vi "Main.vi"(11 "Module Admin":refnum<class "Delacor_lib_QMH_Module Admin.lvclass">) -> ()   [LabVIEW 2020, in "My Singleton Module.lvlib"]
doc: "This template is based off of the Queued Message Handler design pattern and the Queued Message Handler project template that ships with LabVIEW.\n\nThe main difference is that the queue is private to this module and communication between modules is performed via Broadcast and Request events.\n\nRequest events are wrapped in public API methods and are handled in the Event Handling Loop (EHL) of this VI. Any module can register for Broadcast events sent by this module. The EHL generates messages based on user interface actions.\n\nThe Message Handling Loop (MHL) processes messages generated by the EHL, or by other messages. The messages are string values, so new messages can be added easily to the Message Cases case structure in the MHL. Each message cluster can also provide an optional value for Message Data, which is a variant that can be converted to whatever message-specific data is required.\n_____\nBased on Delacor QMH Project Template 5.0.0.82."
uses:
  My Singleton Module.lvlib
  <vilib>/Delacor/Delacor QMH/Libraries/Module Admin_class/Delacor_lib_QMH_Module Admin.lvclass
  Module Data--cluster.ctl
  Do Something Argument--cluster.ctl
  <vilib>/Delacor/Delacor QMH/Libraries/Message Queue_class/Delacor_lib_QMH_Message Queue.lvclass/Delacor_lib_QMH_Message Queue.ctl
  Do Something Else Argument--cluster.ctl
  Do Something Else and Wait for Reply Argument--cluster.ctl
  Do Something Else and Wait (Reply Payload)--cluster.ctl
  Stop Argument--cluster.ctl
  <vilib>/Delacor/Delacor QMH/Libraries/Module Admin_class/Delacor_lib_QMH_Module Admin.lvclass/Delacor_lib_QMH_Module Admin.ctl
  <vilib>/Utility/miscctls.llb/LVPointTypeDef.ctl
  <vilib>/Delacor/Delacor QMH/Libraries/Message Queue_class/Delacor_lib_QMH_Enqueue Message (Single).vi
  <vilib>/Delacor/Delacor QMH/Libraries/Module Admin_class/Delacor_lib_QMH_Get External Launch.vi
  <vilib>/Utility/error.llb/Error Cluster From Error Code.vi
  <vilib>/ErrorRing/Error Ring.xnode
  <vilib>/Delacor/Delacor QMH/Libraries/Message Queue_class/Delacor_lib_QMH_Message Queue.lvclass
panel:
  in  "Simulate MHL Error":bool
  in  "Simulate EHL Error":bool
  out "error out":errorcluster
  out "X":dbl
  out "Status":string
  in  "Do Something Else <Replace Me>":bool
  in  "Do Something <Replace Me>":bool
  # "These controls have associated \"Value Changed\" events configured in the Event Structure on the diagram.\n\nReplace them (and reconfigure the Event Structure) with the controls you need for your application. \n\nOther QMH Modules communicate with this Module via its Public API (wrappers for its Request Events).\n\nThis Module communicates with other Modules via its Broadcast Events.\nAny module that wants to get these messages, just registers for this module's Broadcast events."
  # "This template is for the Delacor Modified Queued Message Handler design pattern.\n\nSee the block diagram for more information on how to use this template."
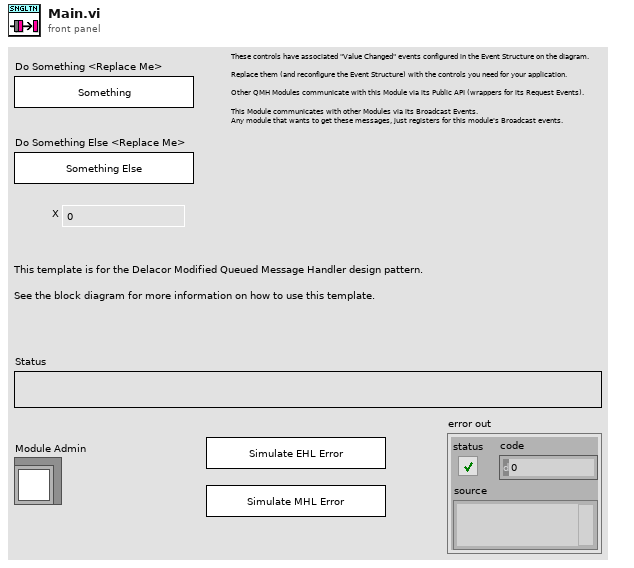
[diagram p1: front panel]
types:
  T1 = typedef "My Singleton Module.lvlib/Request Events--cluster.ctl" = cluster{"Stop Module":refnum<user-event>, "Do Something":refnum<user-event>, "Do Something Else":refnum<user-event>, "Do Something Else and Wait for Reply":refnum<user-event>, "Show Panel":refnum<user-event>, "Hide Panel":refnum<user-event>, "Get Module Execution Status":refnum<user-event>, "Show Diagram":refnum<user-event>}
  T2 = typedef "My Singleton Module.lvlib/Module Data--cluster.ctl" = cluster{"Status":string}
  T3 = typedef "My Singleton Module.lvlib/Do Something Argument--cluster.ctl" = cluster{"Do Something Msg":string}
  T4 = typedef "My Singleton Module.lvlib/Do Something Else Argument--cluster.ctl" = cluster{"Do Something Else Msg":string, "X":dbl}
  T5 = typedef "My Singleton Module.lvlib/Do Something Else and Wait for Reply Argument--cluster.ctl" = cluster{"Do Something Else Msg":string, "X":dbl, "Wait Notifier":refnum<notifier>, "wait for reply":bool}
  T6 = enum32{"invalid lock state", "Not Locked", "Locked (No Password)", "Password-protected"}
  T7 = typedef "My Singleton Module.lvlib/Stop Argument--cluster.ctl" = cluster{"Origin":string, "Exit via Stop Module Req?":bool, "Wait for Module to stop?":bool}
  T8 = typedef "LVPointTypeDef.ctl" = cluster{"Horizontal":i16, "Vertical":i16}
  T9 = enum32{"Invalid", "Standard", "Closed", "Hidden", "Minimized", "Maximized"}
  T10 = typedef "My Singleton Module.lvlib/Do Something Else and Wait (Reply Payload)--cluster.ctl" = cluster{"Value":dbl, "error":errorcluster}
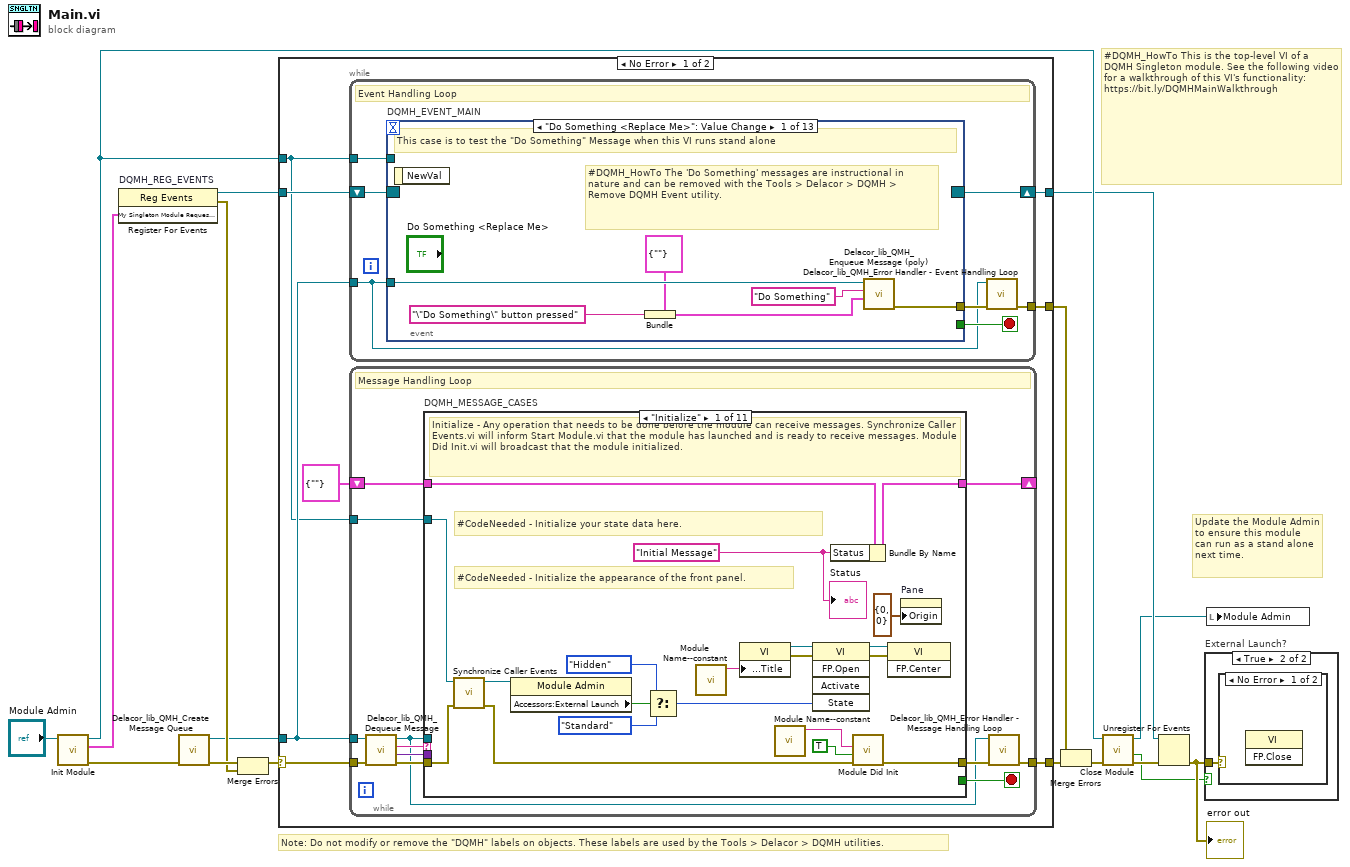
[diagram p0: block diagram]
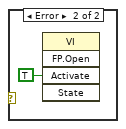
[diagram p3: hidden frame]
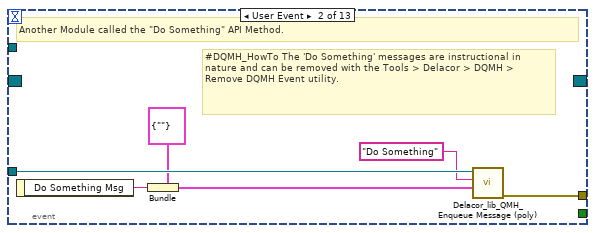
[diagram p4: hidden frame]
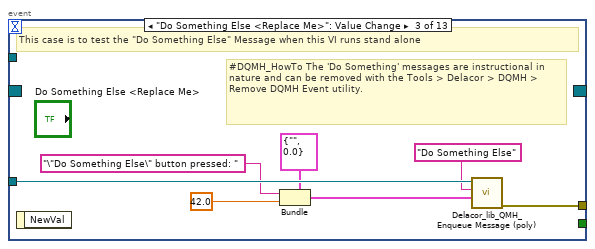
[diagram p5: hidden frame]
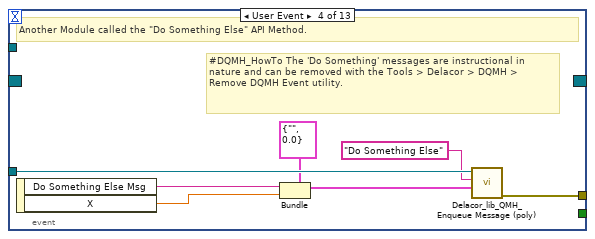
[diagram p6: hidden frame]
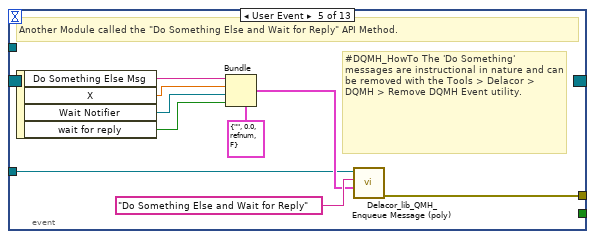
[diagram p7: hidden frame]
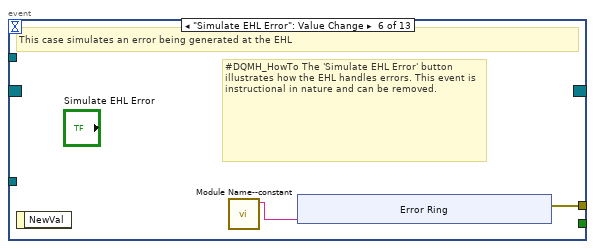
[diagram p8: hidden frame]
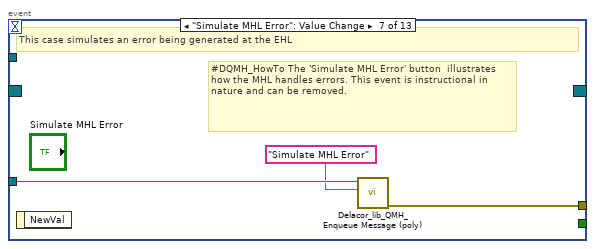
[diagram p9: hidden frame]
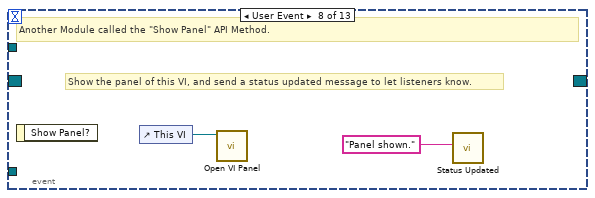
[diagram p10: hidden frame]
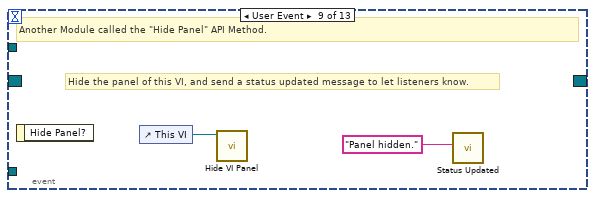
[diagram p11: hidden frame]
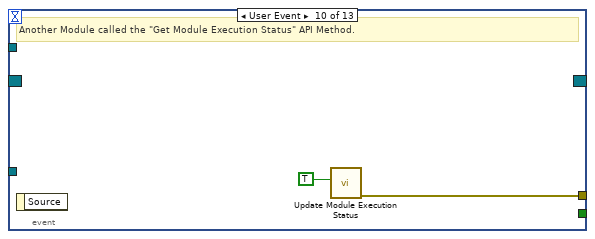
[diagram p12: hidden frame]
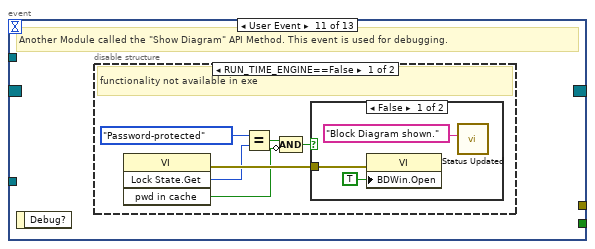
[diagram p13: hidden frame]
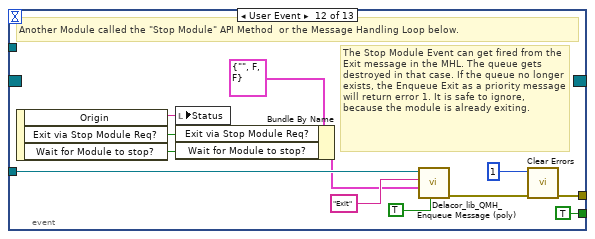
[diagram p16: hidden frame]
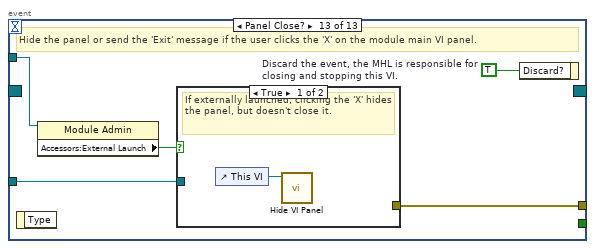
[diagram p17: hidden frame]
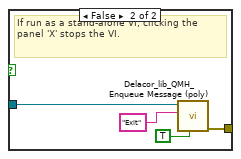
[diagram p18: hidden frame]
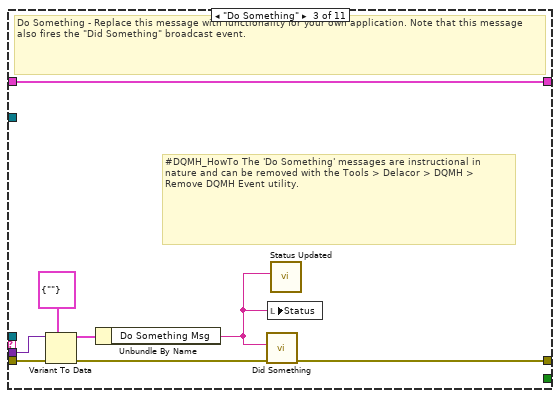
[diagram p20: hidden frame]
diagram:
  # "#DQMH_HowTo This is the top-level VI of a DQMH Singleton module. See the following video for a walkthrough of this VI's functionality: https://bit.ly/DQMHMainWalkthrough"
  # "Note: Do not modify or remove the \"DQMH\" labels on objects. These labels are used by the Tools > Delacor > DQMH utilities."
  # "Update the Module Admin to ensure this module can run as a stand alone next time."
  n1 = call "Init Module.vi"("Singleton Module Admin in"="Module Admin") -> ("error out"=w16:errorcluster, "My Singleton Module Request Events"=w5:T1, "Singleton Module Admin out"=w8:refnum<class "Delacor_lib_QMH_Module Admin.lvclass">)  [unwired: 8 in]
  n2 = register-events "DQMH_REG_EVENTS"(w5) -> (reference out=w6:refnum<event-registration>, error out=w9:errorcluster)  [unwired: 2 in]
  n3 = call <vilib>:"Delacor_lib_QMH_Create Message Queue.vi"("error in (no error)"=w16) -> ("error out"=w11:errorcluster, "Message Queue"=w4:refnum<class "Delacor_lib_QMH_Message Queue.lvclass">)  [unwired: 9 in]
  n4 = Merge Errors(w11, w9) -> (w10:errorcluster)
  n5 = case shown="No Error" w10 {
    selector: w10 -> [w23 w264]
    tunnel: [w25 w263] -> w17
    tunnel: [w22 w269] -> w7
    tunnel: w6 -> [w20 w269]
    tunnel: w4 -> [w19 w262]
    tunnel: [w24 _] -> w14
    tunnel: w8 -> [w18 w265]
    frame No Error {
      n6 = while {
        tunnel: w19 -> [w26]
        shift-right: [w29] -> w22
        shift-left: w20 -> [w30]
        tunnel: [w31] -> w24
        tunnel: w18 -> [w27]
        stop <- w28 stop-if-true
        # "Event Handling Loop"
        n7 = event "DQMH_EVENT_MAIN" shown="[0] \"Do Something <Replace Me>\": Value Change" {
          selector: w30 -> [_ _ _ _ _ _ _ _ _ _ _ _ _]
          dyn-events: [_ _ _ _ _ _ _ _ _ _ _ _ _] -> w29
          timeout: _ -> [_ _ _ _ _ _ _ _ _ _ _ _ _]
          tunnel: [_ _ _ _ _ _ _ _ _ _ _ TRUE ("Discard?") _] -> w28
          tunnel: w26 -> [w37 w43 w50 w57 w60 _ w78 _ _ _ _ w102 w109]
          tunnel: [w38 w44 w51 w58 w67 w69 w79 _ _ w85 _ w105 w111] -> w32
          tunnel: w27 -> [_ _ _ _ _ _ _ _ _ _ _ _ w108]
          event "Do Something <Replace Me>": Value Change {
            # "#DQMH_HowTo The 'Do Something' messages are instructional in nature and can be removed with the Tools > Delacor > DQMH > Remove DQMH Event utility."
            # "This case is to test the \"Do Something\" Message when this VI runs stand alone"
            n8 = event-data() -> ()  [unwired: 1 in, 1 out]
            n9 = Bundle(cluster=T3 {"Do Something Msg"=""} ("Do Something Argument"), "Do Something Msg"="\"Do Something\" button pressed" ("\"Do Something\" button pressed")) -> (w33:T3)
            n10 = call-poly <vilib>:"Delacor_lib_QMH_Enqueue Message (poly).vi"("Message Data"=w33, "Message"="Do Something", "Message Queue in"=w37) -> ("error out"=w38:errorcluster)  [unwired: 7 in, 1 out]
          }
          event User Event {
            # "#DQMH_HowTo The 'Do Something' messages are instructional in nature and can be removed with the Tools > Delacor > DQMH > Remove DQMH Event utility."
            # "Another Module called the \"Do Something\" API Method."
            n11 = event-data() -> ("Do Something Msg"=w40:string)  [unwired: 1 in]
            n12 = Bundle(cluster=T3 {"Do Something Msg"=""} ("Do Something Argument"), "Do Something Msg"=w40) -> (w39:T3)
            n13 = call-poly <vilib>:"Delacor_lib_QMH_Enqueue Message (poly).vi"("Message Data"=w39, "Message"="Do Something", "Message Queue in"=w43) -> ("error out"=w44:errorcluster)  [unwired: 7 in, 1 out]
          }
          event "Do Something Else <Replace Me>": Value Change {
            # "#DQMH_HowTo The 'Do Something' messages are instructional in nature and can be removed with the Tools > Delacor > DQMH > Remove DQMH Event utility."
            # "This case is to test the \"Do Something Else\" Message when this VI runs stand alone"
            n14 = event-data() -> ()  [unwired: 1 in, 1 out]
            n15 = Bundle(cluster=T4 {"Do Something Else Msg"="", "X"=0.0} ("Do Something Else Argument"), "Do Something Else Msg"="\"Do Something Else\" button pressed: " ("\"Do Something Else\" button pressed"), "X"=42.0) -> (w47:T4)
            n16 = call-poly <vilib>:"Delacor_lib_QMH_Enqueue Message (poly).vi"("Message Data"=w47, "Message"="Do Something Else", "Message Queue in"=w50) -> ("error out"=w51:errorcluster)  [unwired: 7 in, 1 out]
          }
          event User Event {
            # "#DQMH_HowTo The 'Do Something' messages are instructional in nature and can be removed with the Tools > Delacor > DQMH > Remove DQMH Event utility."
            # "Another Module called the \"Do Something Else\" API Method."
            n17 = event-data() -> ("Do Something Else Msg"=w53:string, "X"=w52:dbl)  [unwired: 1 in]
            n18 = Bundle(cluster=T4 {"Do Something Else Msg"="", "X"=0.0} ("Do Something Else Argument"), "Do Something Else Msg"=w53, "X"=w52) -> (w54:T4)
            n19 = call-poly <vilib>:"Delacor_lib_QMH_Enqueue Message (poly).vi"("Message Data"=w54, "Message"="Do Something Else", "Message Queue in"=w57) -> ("error out"=w58:errorcluster)  [unwired: 7 in, 1 out]
          }
          event User Event {
            # "#DQMH_HowTo The 'Do Something' messages are instructional in nature and can be removed with the Tools > Delacor > DQMH > Remove DQMH Event utility."
            # "Another Module called the \"Do Something Else and Wait for Reply\" API Method."
            n20 = event-data() -> ("Do Something Else Msg"=w63:string, "X"=w62:dbl, "Wait Notifier"=w61:refnum<notifier>, "wait for reply"=w59:bool)  [unwired: 1 in]
            n21 = Bundle(cluster=T5 {"Do Something Else Msg"="", "X"=0.0, "Wait Notifier"=refnum, "wait for reply"=FALSE} ("Do Something Else and Wait for Reply Argument"), "Do Something Else Msg"=w63, "X"=w62, "Wait Notifier"=w61, "wait for reply"=w59) -> (w64:T5)
            n22 = call-poly <vilib>:"Delacor_lib_QMH_Enqueue Message (poly).vi"("Message Data"=w64, "Message"="Do Something Else and Wait for Reply", "Message Queue in"=w60) -> ("error out"=w67:errorcluster)  [unwired: 7 in, 1 out]
          }
          event "Simulate EHL Error": Value Change {
            # "#DQMH_HowTo The 'Simulate EHL Error' button  illustrates how the EHL handles errors. This event is instructional in nature and can be removed."
            # "This case simulates an error being generated at the EHL"
            n23 = event-data() -> ()  [unwired: 1 in, 1 out]
            n24 = call "Module Name--constant.vi"() -> ("Module Name"=w68:string)  [unwired: 11 in]
            n25 = xnode "Error Ring"("parameter 0"=w68) -> ("error out"=w69:errorcluster)
          }
          event "Simulate MHL Error": Value Change {
            # "#DQMH_HowTo The 'Simulate MHL Error' button  illustrates how the MHL handles errors. This event is instructional in nature and can be removed."
            # "This case simulates an error being generated at the EHL"
            n26 = event-data() -> ()  [unwired: 1 in, 1 out]
            n27 = call-poly <vilib>:"Delacor_lib_QMH_Enqueue Message (poly).vi"("Message"="Simulate MHL Error", "Message Queue in"=w78) -> ("error out"=w79:errorcluster)  [unwired: 8 in, 1 out]
          }
          event User Event {
            # "Show the panel of this VI, and send a status updated message to let listeners know."
            # "Another Module called the \"Show Panel\" API Method."
            n28 = event-data() -> ()  [unwired: 1 in, 1 out]
            n29 = control-ref of="This VI"() -> (w81:refnum<vi>)
            n30 = call "Open VI Panel.vi"("VI"=w81) -> ()  [unwired: 10 in, 1 out]
            n31 = call "Status Updated.vi"("Status"="Panel shown." ("format string")) -> ()  [unwired: 10 in, 1 out]
          }
          event User Event {
            # "Hide the panel of this VI, and send a status updated message to let listeners know."
            # "Another Module called the \"Hide Panel\" API Method."
            n32 = event-data() -> ()  [unwired: 1 in, 1 out]
            n33 = control-ref of="This VI"() -> (w83:refnum<vi>)
            n34 = call "Hide VI Panel.vi"("VI"=w83) -> ()  [unwired: 10 in, 1 out]
            n35 = call "Status Updated.vi"("Status"="Panel hidden." ("format string")) -> ()  [unwired: 10 in, 1 out]
          }
          event User Event {
            # "Another Module called the \"Get Module Execution Status\" API Method."
            n36 = event-data() -> ()  [unwired: 1 in, 1 out]
            n37 = call "Update Module Execution Status.vi"("Running?"=TRUE) -> ("error out"=w85:errorcluster)  [unwired: 10 in]
          }
          event User Event {
            # "Another Module called the \"Show Diagram\" API Method. This event is used for debugging."
            n38 = event-data() -> ()  [unwired: 1 in, 1 out]
            n39 = disable-structure shown="RUN_TIME_ENGINE==False" {
              frame condition #0 (active) {
                # "functionality not available in exe"
                n40 = invoke class="VI" method="Lock State.Get"() -> (error out=w91:errorcluster, "Get Lock State"=w90:T6, "pwd in cache"=w87:bool)  [unwired: 4 in, 1 out]
                n41 = Equal?(x=T6."Password-protected", y=w90) -> (x = y?=w88:bool)
                n42 = Compound Arithmetic op=AND(w88, invert w87) -> (w86:bool)
                n43 = case shown="False" w86 {
                  tunnel: w91 -> [w94 _]
                  frame False {
                    n44 = property class="VI"(error in=w94, "BDWin.Open"=TRUE ("Block Diagram Window:Open")) -> ()  [unwired: 1 in, 2 out]
                    n45 = call "Status Updated.vi"("Status"="Block Diagram shown." ("format string")) -> ()  [unwired: 10 in, 1 out]
                  }
                  frame True {
                    # "Password-protected VI, and the password is not in the cache. Do not show the diagram."
                  }
                }
              }
              frame condition #1 {
              }
            }
          }
          event User Event {
            # "The Stop Module Event can get fired from the Exit message in the MHL. The queue gets destroyed in that case. If the queue no longer exists, the Enqueue Exit as a priority message will return error 1. It is safe to ignore, because the module is already exiting."
            # "Another Module called the \"Stop Module\" API Method  or the Message Handling Loop below."
            n46 = event-data() -> ("Origin"=w101:string, "Exit via Stop Module Req?"=w97:bool, "Wait for Module to stop?"=w96:bool)  [unwired: 1 in]
            n47 = local write "Status"(w101) -> ()
            n48 = Bundle By Name(cluster=T7 {"Origin"="", "Exit via Stop Module Req?"=FALSE, "Wait for Module to stop?"=FALSE} ("Stop Argument"), "Exit via Stop Module Req?"=w97, "Wait for Module to stop?"=w96) -> (w95:T7)
            n49 = call-poly <vilib>:"Delacor_lib_QMH_Enqueue Message (poly).vi"("Priority Message? (F)"=TRUE, "Message Data"=w95, "Message"="Exit", "Message Queue in"=w102) -> ("error out"=w106:errorcluster)  [unwired: 6 in, 1 out]
            n50 = call <vilib>:"Clear Errors.vi"("error in (no error)"=w106, "specific error code to clear (0: all)"=1) -> ("error out"=w105:errorcluster)  [unwired: 4 in, 1 out]
          }
          event Panel Close? {
            w110 = TRUE  # Discard the event, the MHL is responsible for closing and stopping this VI.
            # "Hide the panel or send the 'Exit' message if the user clicks the 'X' on the module main VI panel."
            n51 = event-data() -> ()  [unwired: 1 in, 1 out]
            n52 = property class="Module Admin"(reference=w108) -> ("Accessors:External Launch"=w107:bool)  [unwired: 1 in, 2 out]
            n53 = case shown="True" w107 {
              tunnel: w109 -> [_ w115]
              tunnel: [_ w116] -> w111
              frame True {
                # "If externally launched, clicking the 'X' hides the panel, but doesn't close it."
                n54 = control-ref of="This VI"() -> (w112:refnum<vi>)
                n55 = call "Hide VI Panel.vi"("VI"=w112) -> ()  [unwired: 10 in, 1 out]
              }
              frame False {
                # "If run as a stand-alone VI, clicking the panel 'X' stops the VI."
                n56 = call-poly <vilib>:"Delacor_lib_QMH_Enqueue Message (poly).vi"("Priority Message? (F)"=TRUE, "Message"="Exit", "Message Queue in"=w115) -> ("error out"=w116:errorcluster)  [unwired: 7 in, 1 out]
              }
            }
            n57 = event-data("Discard?"=w110) -> ()  [unwired: 1 in, 1 out]
          }
        }
        n58 = call-dynamic "Delacor_lib_QMH_Error Handler - Event Handling Loop.vi"("error in (no error)"=w32, "Message Queue in"=w26) -> ("dup error in"=w31:errorcluster)  [unwired: 8 in, 1 out]
      }
      n59 = while {
        tunnel: w19 -> [w119]
        shift-right: [w123] -> _
        shift-left: T2 {"Status"=""} ("Data Cluster") -> [w124]
        tunnel: w23 -> [w127]
        tunnel: [w125] -> w25
        tunnel: w18 -> [w117]
        stop <- w122 stop-if-true
        # "Message Handling Loop"
        n60 = call-dynamic "Delacor_lib_QMH_Dequeue Message.vi"("error in (no error)"=w127, "Message Queue in"=w119) -> ("error out"=w126:errorcluster, "Message Data"=w120:variant, "Message"=w121:string, "Message Queue out"=w118:refnum<class "Delacor_lib_QMH_Message Queue.lvclass">)  [unwired: 6 in]
        n61 = case "DQMH_MESSAGE_CASES" shown="\"Initialize\"" w121 {
          selector: w121 -> [_ _ _ _ _ _ _ _ _ _ w249]
          tunnel: w118 -> [_ _ _ _ _ _ _ _ w219 w241 _]
          tunnel: w126 -> [w146 w150 w158 w167 w186 w201 w203 w208 w226 w247 w251]
          tunnel: [w144 w150 w156 w166 w185 w200 w203 w207 w222 w244 w252] -> w128
          tunnel: w124 -> [w135 w149 w155 w165 w183 w199 w202 w205 w221 w240 w250]
          tunnel: [w134 w149 w155 w165 w183 w199 w202 w205 w221 w240 w250] -> w123
          tunnel: [_ _ _ _ _ _ _ _ _ w239 _] -> w122
          tunnel: w120 -> [_ _ w154 w162 w180 _ _ _ w220 w238 _]
          tunnel: w117 -> [w136 _ _ _ _ _ _ _ w218 w233 _]
          frame "Initialize" {
            w129 = "Initial Message" ("Initial Message")
            # "#CodeNeeded - Initialize the appearance of the front panel."
            # "#CodeNeeded - Initialize your state data here."
            # "Initialize - Any operation that needs to be done before the module can receive messages. Synchronize Caller Events.vi will inform Start Module.vi that the module has launched and is ready to receive messages. Module Did Init.vi will broadcast that the module initialized."
            n62 = call "Synchronize Caller Events.vi"("error in (no error)"=w146, "Singleton Module Admin in"=w136) -> ("error out"=w145:errorcluster, "Singleton Module Admin out"=w131:refnum<class "Delacor_lib_QMH_Module Admin.lvclass">)  [unwired: 8 in]
            n63 = property class="Module Admin"(reference=w131) -> ("Accessors:External Launch"=w140:bool)  [unwired: 1 in, 2 out]
            n64 = Select(t=T9."Hidden" ("State"), s=w140, f=T9."Standard" ("State")) -> (s? t:f=w137:T9)
            n65 = call "Module Name--constant.vi"() -> ("Module Name"=w143:string)  [unwired: 11 in]
            n66 = property class="VI"("Front Panel.Title"=w143) -> (reference out=w142:refnum<vi>, error out=w148:errorcluster)  [unwired: 2 in]
            n67 = call "Module Name--constant.vi"() -> ("Module Name"=w132:string)  [unwired: 11 in]
            n68 = invoke class="VI" method="FP.Open"(reference=w142, error in=w148, "State"=w137) -> (reference out=w141:refnum<vi>, error out=w147:errorcluster)  [unwired: 2 in, 3 out]
            n69 = Bundle By Name(cluster=w135, "Status"=w129) -> (w134:T2)
            n70 = call "Module Did Init.vi"("error in (no error)"=w145, "Initialized?"=TRUE, "Origin"=w132) -> ("error out"=w144:errorcluster)  [unwired: 8 in]
            n71 = invoke class="VI" method="FP.Center"(reference=w141, error in=w147) -> ()  [unwired: 1 in, 3 out]
            n72 = property on="Pane" class="Pane"("Origin"=T8 {"Horizontal"=0, "Vertical"=0}) -> ()  [unwired: 2 in, 2 out]
            "Status" <- w129
          }
          frame "--- Module Specific ---" {
            # "Separator -- The following cases handle messages specific to this Module."
          }
          frame "Do Something" {
            # "#DQMH_HowTo The 'Do Something' messages are instructional in nature and can be removed with the Tools > Delacor > DQMH > Remove DQMH Event utility."
            # "Do Something - Replace this message with functionality for your own application. Note that this message also fires the \"Did Something\" broadcast event."
            n73 = Variant To Data(error in=w158, type=T3 {"Do Something Msg"=""} ("Do Something Argument"), Variant=w154) -> (data=w153:T3, error out=w157:errorcluster)
            n74 = Unbundle By Name(w153) -> ("Do Something Msg"=w151:string)
            n75 = call "Did Something.vi"("error in (no error)"=w157, "Did Something Msg"=w151) -> ("error out"=w156:errorcluster)  [unwired: 9 in]
            n76 = local write "Status"(w151) -> ()
            n77 = call "Status Updated.vi"("Status"=w151) -> ()  [unwired: 10 in, 1 out]
          }
          frame "Do Something Else" {
            # "#DQMH_HowTo The 'Do Something' messages are instructional in nature and can be removed with the Tools > Delacor > DQMH > Remove DQMH Event utility."
            # "Do Something Else - Replace this message with functionality for your own application."
            n78 = Variant To Data(error in=w167, type=T4 {"Do Something Else Msg"="", "X"=0.0} ("Do Something Else Argument"), Variant=w162) -> (data=w163:T4, error out=w166:errorcluster)
            n79 = Unbundle By Name(w163) -> ("Do Something Else Msg"=w161:string, "X"=w160:dbl)
            "X" <- w160
            n80 = Format Into String(initial string=w161, w160) -> (resulting string=w159:string)  [unwired: 2 in, 1 out]
            n81 = local write "Status"(w159) -> ()
            n82 = call "Status Updated.vi"("Status"=w159) -> ()  [unwired: 10 in, 1 out]
          }
          frame "Do Something Else and Wait for Reply" {
            w175 = "X(%.2f)+Offset(%.2f)=%.2f"  # status message format string
            # "#DQMH_HowTo The 'Do Something' messages are instructional in nature and can be removed."
            # "Send back X with a random offset"
            # "Do Something Else and Wait for Reply - Replace this message with functionality for your own application. Note that this message must fire a notifier to let callers know it has finished execution, and it returns an error if the 'Value' is negative."
            n83 = Random Number (0-1)() -> (number: 0 to 1=w177:dbl)
            n84 = Variant To Data(error in=w186, type=T5 {"Do Something Else Msg"="", "X"=0.0, "Wait Notifier"=refnum, "wait for reply"=FALSE} ("Do Something Else and Wait for Reply Argument"), Variant=w180) -> (data=w181:T5, error out=w184:errorcluster)
            n85 = Unbundle By Name(w181) -> ("Wait Notifier"=w168:refnum<notifier>, "Do Something Else Msg"=w179:string, "X"=w176:dbl, "wait for reply"=w172:bool)
            n86 = Add(x=w177, y=w176) -> (x+y=w171:dbl)
            n87 = local write "X"(w176) -> ()
            n88 = Less Than 0?(x=w171) -> (x < 0?=w174:bool)
            n89 = Format Into String(format string=w175, initial string=w179, w176, w177, w171) -> (resulting string=w173:string)  [unwired: 1 in, 1 out]
            n90 = case shown="True" w174 {
              tunnel: [_ w193] -> w169
              frame False {
              }
              frame True {
                n91 = xnode "Error Ring"() -> ("error out"=w193:errorcluster)
              }
            }
            n92 = Bundle By Name(cluster=T10 {"Value"=0.0, "error"={"status"=FALSE, "code"=0, "source"=""}} ("notification"), "error"=w169, "Value"=w171) -> (w170:T10)
            n93 = local write "Status"(w173) -> ()
            n94 = call "Status Updated.vi"("Status"=w173) -> ()  [unwired: 10 in, 1 out]
            n95 = case shown="True" w172 {
              tunnel: w170 -> [_ w189]
              tunnel: w168 -> [_ w188]
              frame False {
              }
              frame True {
                # "Simulate an operation that requires a wait."
                n96 = flat-sequence {
                  tunnel: w189 -> [w192]
                  tunnel: w188 -> [w191]
                  tunnel: w187 -> [_]
                  frame #0 {
                    n97 = Send Notification(notification=w192, notifier=w191) -> ()  [unwired: 1 in, 2 out]
                  }
                }
                n98 = Wait (ms)(milliseconds to wait=u32 1000) -> (millisecond timer value=w187:u32)
              }
            }
            n99 = Merge Errors(w184, w169) -> (w185:errorcluster)
          }
          frame "---Copy This Frame---" {
            # "Duplicate this frame when creating new messages.  Change this comment in the duplicated frame to describe this message."
            n100 = Merge Errors(w201) -> (w200:errorcluster)
          }
          frame "--- Exit and Error Handling---" {
            # "Separator - The following cases handle errors and exit messages."
          }
          frame "Simulate MHL Error" {
            # "#DQMH_HowTo The 'Simulate MHL Error' button  illustrates how the MHL handles errors. This event is instructional in nature and can be removed."
            # "Simulate an error occurring at the MHL"
            n101 = call "Module Name--constant.vi"() -> ("Module Name"=w204:string)  [unwired: 11 in]
            n102 = xnode "Error Ring"("parameter 0"=w204) -> ("error out"=w206:errorcluster)
            n103 = Merge Errors(w208, w206) -> (w207:errorcluster)
          }
          frame "Error" {
            # "#CodeRecommended - If you ever change the name of this \"Error\" message, you'll need to update the name in the Check Loop Error.vi as well."
            # "#CodeRecommended - If the module is running in standalone mode (External Launch = FALSE), this code will pop up an error dialog and call the 'Exit' message if an error occurs. Add more fine-grained error handling here."
            # "Error - Check the error message data and respond accordingly. This message is sent by the \"Error Handler\" VIs at the end of each loop in this application."
            n104 = property class="Module Admin"(reference=w218) -> ("Accessors:External Launch"=w217:bool)  [unwired: 1 in, 2 out]
            n105 = Variant To Data(error in=w226, type=errorcluster {"status"=FALSE, "code"=0, "source"=""} ("error constant"), Variant=w220) -> (data=w227:errorcluster, error out=w224:errorcluster)
            n106 = call "Module Name--constant.vi"() -> ("Module Name"=w216:string)  [unwired: 11 in]
            n107 = call "Error Reported.vi"("Additional Information"=w216, "Error"=w227) -> ()  [unwired: 9 in, 1 out]
            n108 = case shown="False" w217 {
              tunnel: [w232 _] -> w223
              tunnel: w219 -> [w230 _]
              tunnel: w227 -> [w231 _]
              frame False {
                # "If the module is running standalone, then pop up an error dialog and call the \"Exit\" message."
                n109 = call <vilib>:"Simple Error Handler.vi"("error in (no error)"=w231) -> ()  [unwired: 4 in, 5 out]
                n110 = call-poly <vilib>:"Delacor_lib_QMH_Enqueue Message (poly).vi"("Priority Message? (F)"=TRUE, "Message"="Exit", "Message Queue in"=w230) -> ("error out"=w232:errorcluster)  [unwired: 7 in, 1 out]
              }
              frame True {
                # "If the module was launched externally, calling the Error Reported broadcast VI is the only action performed by the \"Error\" message. The module's caller can then process the error appropriately."
              }
            }
            n111 = Merge Errors(w224, w223) -> (w222:errorcluster)
            n112 = local write "error out"(w222) -> ()
          }
          frame "Exit" {
            w237 = 91  # 91: not all Exit messages will have an argument
            w239 = TRUE  # Stop the VI
            # "Release the message queue reference"
            # "#CodeNeeded - Add any required cleanup code here"
            # "Exit - Exit the application."
            n113 = Variant To Data(error in=w247, type=T7 {"Origin"="", "Exit via Stop Module Req?"=FALSE, "Wait for Module to stop?"=FALSE} ("Stop Argument"), Variant=w238) -> (data=w235:T7, error out=w243:errorcluster)
            n114 = call <vilib>:"Clear Errors.vi"("error in (no error)"=w243, "specific error code to clear (0: all)"=w237) -> ("error out"=w246:errorcluster)  [unwired: 4 in, 1 out]
            n115 = control-ref of="This VI"() -> (w234:refnum<vi>)
            n116 = call-dynamic "Delacor_lib_QMH_Release Message Queue.vi"("error in (no error)"=w246, "Message Queue"=w241) -> ("error out"=w245:errorcluster)  [unwired: 9 in]
            n117 = call "Handle Exit.vi"("Stop Argument"=w235, "Admin in"=w233, "VI reference"=w234) -> ("error out"=w242:errorcluster)  [unwired: 7 in, 1 out]
            n118 = Merge Errors(w245, w242) -> (w244:errorcluster)
          }
          frame Default {
            # "'Default' case only runs if there is a message that isn't defined in any of the other cases.  Output a programming error."
            n119 = call "Module Name--constant.vi"() -> ("Module Name"=w248:string)  [unwired: 11 in]
            n120 = xnode "Error Ring"("parameter 0"=w249, "parameter 1"=w248) -> ("error out"=w253:errorcluster)
            n121 = Merge Errors(w251, w253) -> (w252:errorcluster)
          }
        }
        n122 = call-dynamic "Delacor_lib_QMH_Error Handler - Message Handling Loop.vi"("error in (no error)"=w128, "Message Queue in"=w118) -> ("dup error in"=w125:errorcluster)  [unwired: 8 in, 1 out]
      }
    }
    frame Error {
      # "Synchronize Caller Events.vi will inform Start Module.vi that the module has launched and will let the code calling Start Module.vi register for broadcasts and would permit the caller receive the broadcast that an error occurred at launch time."
      n123 = call-dynamic "Delacor_lib_QMH_Release Message Queue.vi"("error in (no error)"=w264, "Message Queue"=w262) -> ("error out"=w263:errorcluster)  [unwired: 9 in]
      n124 = call "Synchronize Caller Events.vi"("Singleton Module Admin in"=w265) -> ("error out"=w270:errorcluster)  [unwired: 9 in, 1 out]
      n125 = call "Module Name--constant.vi"() -> ("Module Name"=w268:string)  [unwired: 11 in]
      n126 = Format Into String(format string="An error occurred during initialization. %s is no longer running.", w268) -> (resulting string=w266:string)  [unwired: 2 in, 1 out]
      n127 = Merge Errors(w263, w270) -> (w271:errorcluster)
      n128 = call "Error Reported.vi"("Additional Information"=w266, "Error"=w271) -> ()  [unwired: 9 in, 1 out]
    }
  }
  n129 = Merge Errors(w14, w17) -> (w13:errorcluster)
  n130 = call "Close Module.vi"("error in (no error)"=w13, "Module Admin in"=w8) -> ("error out"=w15:errorcluster, "External Launch"=w1:bool, "Module Admin out"=w2:refnum<class "Delacor_lib_QMH_Module Admin.lvclass">)  [unwired: 7 in]
  n131 = Unregister For Events(event registration refnum=w7, error in=w15) -> (error out=w12:errorcluster)
  "error out" <- w12
  n132 = case "External Launch?" shown="True" w1 {
    tunnel: w12 -> [_ w272]
    frame False {
    }
    frame True {
      n133 = case shown="No Error" w272 {
        frame No Error {
          n134 = invoke class="VI" method="FP.Close"() -> ()  [unwired: 3 in, 3 out]
        }
        frame Error {
          n135 = invoke class="VI" method="FP.Open"("Activate"=TRUE ("Activate?")) -> ()  [unwired: 4 in, 5 out]
        }
      }
    }
  }
  n136 = local write "Module Admin"(w2) -> ()
